vi "Memory.Pointer.Error Handling.Out of Range.vi"(5 "parameter":T1, 7 "source vi name":string, 8 "error in (no error)":errorcluster, 10 "value":u64 format="%d bytes", 11 "pointer in":refnum<class "Memory.Pointer.lvclass">) -> (0 "error out":errorcluster, 3 "pointer out":refnum<class "Memory.Pointer.lvclass">)   [LabVIEW 2016, in "Memory Manager.lvlib" / "Memory.Pointer.lvclass"]
uses:
  Memory.Pointer.lvclass
  Pointer.Void/Typedefs/Memory.Pointer.Parameters.ctl
  Pointer.Void/Typedefs/Memory.Pointer.Errors.ctl
  Memory.Pointer.lvclass/Memory.Pointer.ctl
  <vilib>/NI/Static Error Handling/VIs/Static Error Handling.Error Cluster Constant (256B).vi
  <vilib>/NI/Static Error Handling/VIs/Static Error Handling.Source Buffer.Write.String.vi
  Accessors/Get Size.vi
  <vilib>/NI/Static Error Handling/VIs/Static Error Handling.Source Buffer.Write.Numeric.Scalar.Base10.vi
  <vilib>/NI/Static Error Handling/VIs/Static Error Handling.Source Buffer.Write.Numeric.Scalar.Base10 (U64).vi
  <vilib>/NI/Static Error Handling/Static Error Handling.lvlib
  Memory Manager.lvlib
  Pointer.Void/Memory.Pointer.Void.lvclass
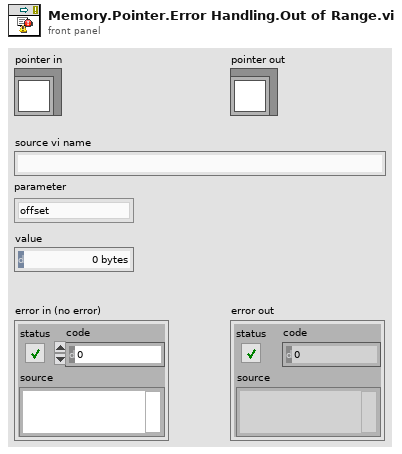
[diagram p1: front panel]
types:
  T1 = typedef "Memory Manager.lvlib/Memory.Pointer.Void.lvclass/Memory.Pointer.Parameters.ctl" = enum16{"offset", "length", "size", "subset"}
  T2 = typedef "Memory Manager.lvlib/Memory.Pointer.Void.lvclass/Memory.Pointer.Errors.ctl" = enum16{"None", "Out of Range"}
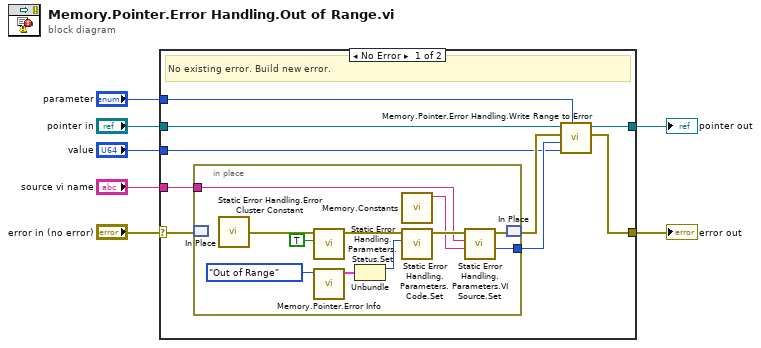
[diagram p0: block diagram]
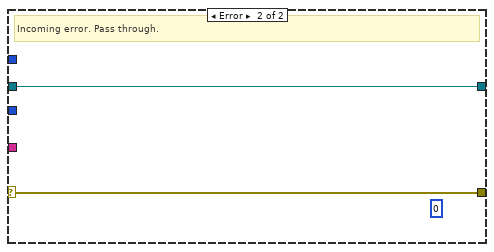
[diagram p2: hidden frame]
diagram:
  n1 = case shown="No Error" "error in (no error)" {
    selector: "error in (no error)" -> [w16 w29]
    tunnel: [w11 w29] -> w4
    tunnel: "value" -> [w8 _]
    tunnel: "source vi name" -> [w15 _]
    tunnel: "parameter" -> [w10 _]
    tunnel: "pointer in" -> [w14 w28]
    tunnel: [w13 w28] -> w1
    frame No Error {
      # "No existing error. Build new error."
      n2 = in-place {
        in-place-border: w15 -> [w24]
        in-place-border: [w20] -> w9
        n3 = in-place-match #1(w16) -> ()  [unwired: 1 out]
        n4 = call-poly <vilib>:"Static Error Handling.Error Cluster Constant.vi"() -> ("error out"=w19:errorcluster)  [unwired: 1 in]
        n5 = call <vilib>:"Static Error Handling.Parameters.Status.Set.vi"("status (T)"=TRUE, "error in"=w19) -> ("error out"=w26:errorcluster)  [unwired: 9 in]
        n6 = call "Memory.Pointer.Error Info.vi"("error (no error)"=Memory.Pointer.Errors."Out of Range" ("error (none)")) -> ("error info"=w18:cluster{"code":i32, "description":string})  [unwired: 10 in]
        n7 = Unbundle(w18) -> ("code"=w17:i32)  [unwired: 1 out]
        n8 = call "Memory.Constants.vi"() -> ("library name"=w23:string)  [unwired: 11 in]
        n9 = call <vilib>:"Static Error Handling.Parameters.Code.Set.vi"("code"=w17, "error in"=w26) -> ("error out"=w25:errorcluster)  [unwired: 9 in]
        n10 = call <vilib>:"Static Error Handling.Parameters.VI Source.Set.vi"("library name (\"\")"=w23, "vi name"=w24, "error in"=w25) -> ("new offset"=w20:i32, "error out"=w21:errorcluster)  [unwired: 7 in]
        n11 = in-place-match #1(w21) -> (w12:errorcluster)
      }
      n12 = call "Memory.Pointer.Error Handling.Write Range to Error.vi"("parameter"=w10, "value"=w8, "offset"=w9, "error in"=w12, "pointer in"=w14) -> ("error out"=w11:errorcluster, "pointer out"=w13:refnum<class "Memory.Pointer.lvclass">)  [unwired: 4 in, 1 out]
    }
    frame Error {
      (unwired) 0 ("new offset")
      # "Incoming error. Pass through."
    }
  }
  "error out" <- w4
  "pointer out" <- w1
